vi "Generate Random Trajectory.vi"(8 "Error In":errorcluster, 10 "Height":u64=100, 11 "Width":u64) -> (0 "Error Out":errorcluster, 2 "Position":T1, 3 "Force":T1)   [LabVIEW 2021, in "Shooting Stars.lvclass"]
uses:
  Shooting Stars.lvclass
  Shooting Stars.lvclass/Shooting Stars.ctl
  Display Utilities/Public/Controls/2D Coordinates.ctl
  Display Utilities/Display Utilities.lvlib
  <vilib>/numeric/Random Number (Range) U64.vi
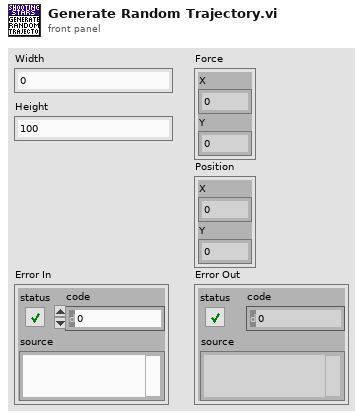
[diagram p1: front panel]
types:
  T1 = typedef "Display Utilities.lvlib/2D Coordinates.ctl" = cluster{"X":i32, "Y":i32}
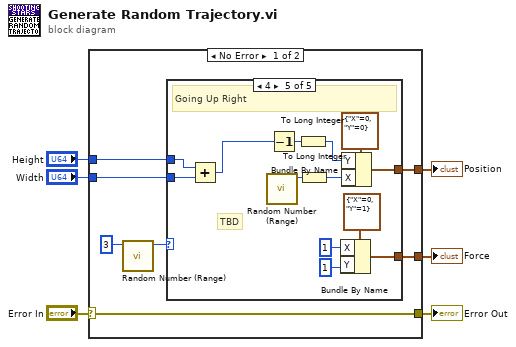
[diagram p0: block diagram]
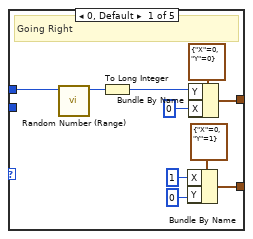
[diagram p2: hidden frame]
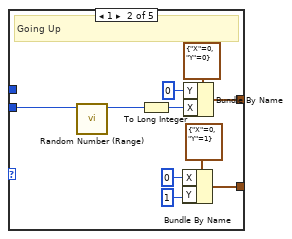
[diagram p3: hidden frame]
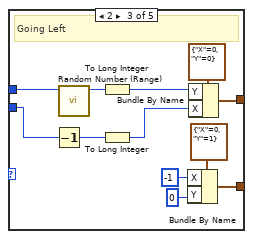
[diagram p4: hidden frame]
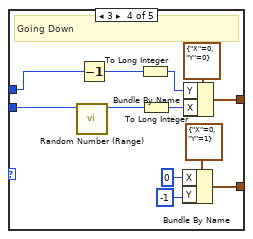
[diagram p5: hidden frame]
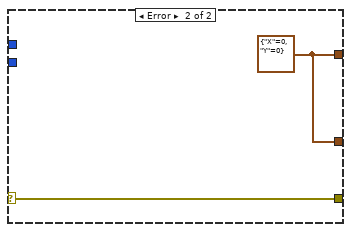
[diagram p6: hidden frame]
diagram:
  n1 = case shown="No Error" "Error In" {
    selector: "Error In" -> [w10 w72]
    tunnel: [w13 w71] -> w6
    tunnel: [w9 w71] -> w5
    tunnel: [w10 w72] -> w3
    tunnel: "Height" -> [w7 _]
    tunnel: "Width" -> [w8 _]
    frame No Error {
      n2 = call-poly <vilib>:"Random Number (Range).vi"("upper bound (100)"=u64 3) -> ("number"=w12:u64)  [unwired: 10 in]
      n3 = case shown="4" w12 {
        tunnel: [w20 w32 w42 w56 w69] -> w13
        tunnel: [w18 w28 w40 w52 w65] -> w9
        tunnel: w8 -> [_ w25 w36 w49 w59]
        tunnel: w7 -> [w14 _ w37 w48 w60]
        frame 0, Default {
          # "Going Right"
          n4 = call-poly <vilib>:"Random Number (Range).vi"("upper bound (100)"=w14) -> ("number"=w15:u64)  [unwired: 10 in]
          n5 = To Long Integer(number=w15) -> (32bit integer=w16:i32)
          n6 = Bundle By Name(cluster=T1 {"X"=0, "Y"=1} ("Position"), "X"=1, "Y"=0) -> (w20:T1)
          n7 = Bundle By Name(cluster=T1 {"X"=0, "Y"=0} ("Position"), "Y"=w16, "X"=0 ("Y")) -> (w18:T1)
        }
        frame 1 {
          # "Going Up"
          n8 = call-poly <vilib>:"Random Number (Range).vi"("upper bound (100)"=w25) -> ("number"=w26:u64)  [unwired: 10 in]
          n9 = To Long Integer(number=w26) -> (32bit integer=w27:i32)
          n10 = Bundle By Name(cluster=T1 {"X"=0, "Y"=1} ("Position"), "X"=0, "Y"=1) -> (w32:T1)
          n11 = Bundle By Name(cluster=T1 {"X"=0, "Y"=0} ("Position"), "Y"=0, "X"=w27) -> (w28:T1)
        }
        frame 2 {
          # "Going Left"
          n12 = Decrement(x=w36) -> (x-1=w35:u64)
          n13 = call-poly <vilib>:"Random Number (Range).vi"("upper bound (100)"=w37) -> ("number"=w38:u64)  [unwired: 10 in]
          n14 = To Long Integer(number=w38) -> (32bit integer=w39:i32)
          n15 = To Long Integer(number=w35) -> (32bit integer=w34:i32)
          n16 = Bundle By Name(cluster=T1 {"X"=0, "Y"=1} ("Position"), "X"=-1, "Y"=0) -> (w42:T1)
          n17 = Bundle By Name(cluster=T1 {"X"=0, "Y"=0} ("Position"), "Y"=w39, "X"=w34) -> (w40:T1)
        }
        frame 3 {
          # "Going Down"
          n18 = call-poly <vilib>:"Random Number (Range).vi"("upper bound (100)"=w49) -> ("number"=w50:u64)  [unwired: 10 in]
          n19 = Decrement(x=w48) -> (x-1=w47:u64)
          n20 = To Long Integer(number=w47) -> (32bit integer=w46:i32)
          n21 = To Long Integer(number=w50) -> (32bit integer=w51:i32)
          n22 = Bundle By Name(cluster=T1 {"X"=0, "Y"=1} ("Position"), "X"=0, "Y"=-1) -> (w56:T1)
          n23 = Bundle By Name(cluster=T1 {"X"=0, "Y"=0} ("Position"), "Y"=w46, "X"=w51) -> (w52:T1)
        }
        frame 4 {
          # "TBD"
          # "Going Up Right"
          n24 = Add(x=w60, y=w59) -> (x+y=w58:u64)
          n25 = call-poly <vilib>:"Random Number (Range).vi"() -> ("number"=w63:u64)  [unwired: 11 in]
          n26 = Decrement(x=w58) -> (x-1=w62:u64)
          n27 = To Long Integer(number=w62) -> (32bit integer=w61:i32)
          n28 = To Long Integer(number=w63) -> (32bit integer=w64:i32)
          n29 = Bundle By Name(cluster=T1 {"X"=0, "Y"=1} ("Position"), "X"=1, "Y"=1) -> (w69:T1)
          n30 = Bundle By Name(cluster=T1 {"X"=0, "Y"=0} ("Position"), "Y"=w61, "X"=w64) -> (w65:T1)
        }
      }
    }
    frame Error {
      w71 = T1 {"X"=0, "Y"=0} ("Position")
    }
  }
  "Force" <- w6
  "Position" <- w5
  "Error Out" <- w3
